vi "PTC-Create Queue Data.vi"(0 "state":T4, 5 "Params":T1, 9 "Acoustic System ID":string) -> (8 "data":T5, 15 "error out":errorcluster)   [LabVIEW 2020]
uses:
  Typedefs/PTC-Queue Data.ctl
  Common VIs/Typedefs/CAL-Stimulus.ctl
  Typedefs/PTC-Response.ctl
  Common VIs/Typedefs/CAL-Endpoint.ctl
  Typedefs/PTC-Parameters.ctl
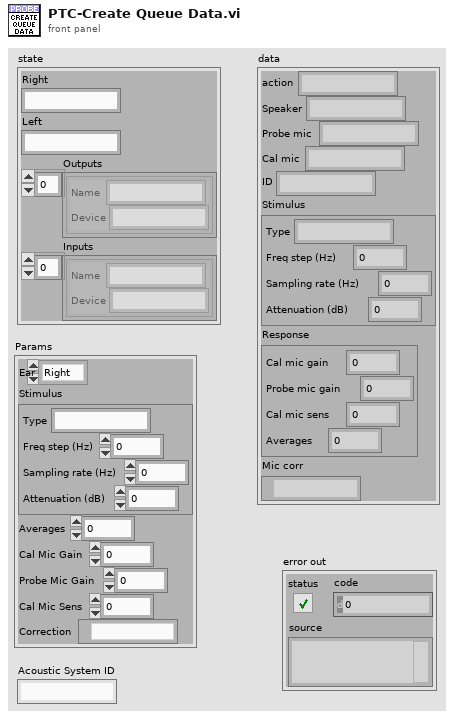
[diagram p1: front panel]
types:
  T1 = typedef "PTC-Parameters.ctl" = cluster{"Ear":enum16{"Right", "Left"}, "Stimulus":T2, "Averages":i32, "Cal Mic Gain":dbl, "Probe Mic Gain":dbl, "Cal Mic Sens":dbl, "Correction":path}
  T2 = typedef "CAL-Stimulus.ctl" = cluster{"Type":string, "Freq step (Hz)":dbl, "Sampling rate (Hz)":dbl, "Attenuation (dB)":dbl}
  T3 = typedef "CAL-Endpoint.ctl" = cluster{"Name":string, "Device":string}
  T4 = cluster{"Right":string, "Left":string, "Outputs":T3[], "Inputs":T3[]}
  T5 = typedef "PTC-Queue Data.ctl" = cluster{"action":string, "Speaker":string, "Probe mic":string, "Cal mic":string, "ID":string, "Stimulus":T2, "Response":T6, "Mic corr":path}
  T6 = typedef "PTC-Response.ctl" = cluster{"Cal mic gain":dbl, "Probe mic gain":dbl, "Cal mic sens":dbl, "Averages":i32}
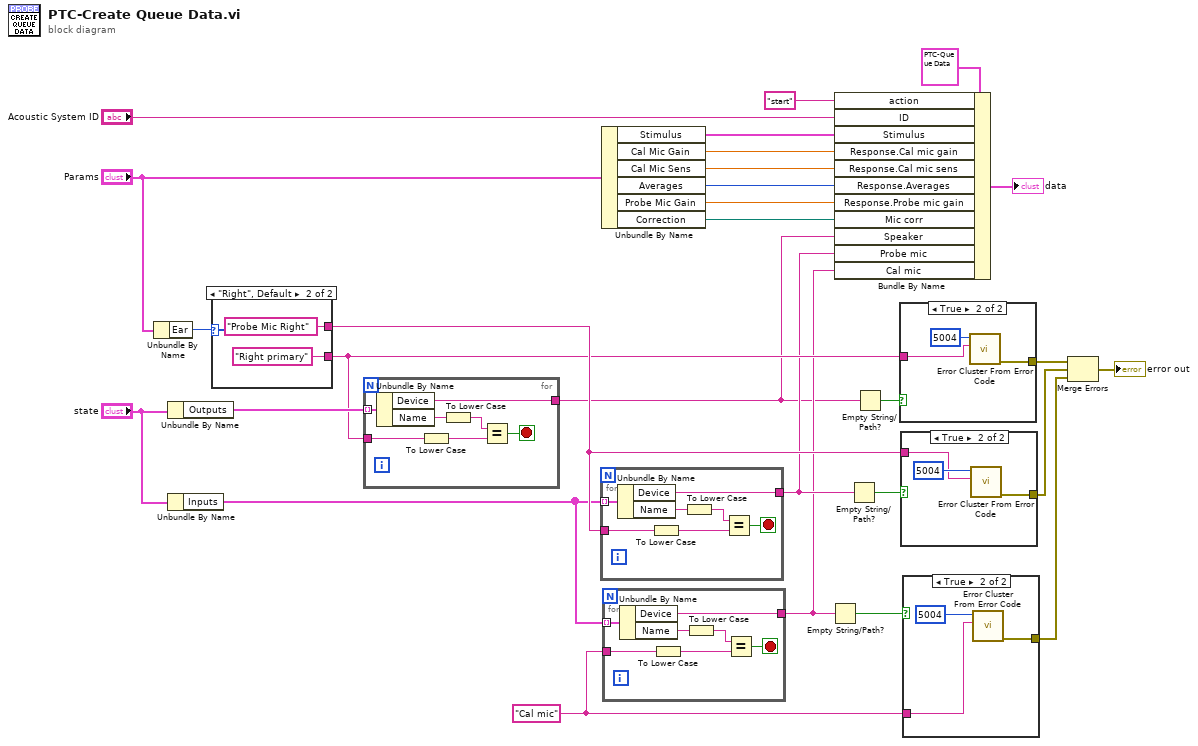
[diagram p0: block diagram]
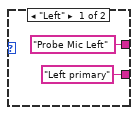
[diagram p3: hidden frame]
diagram:
  w4 = "Cal mic"
  n1 = Unbundle By Name("Params") -> ("Ear"=w24:enum16{"Right", "Left"})
  n2 = Unbundle By Name("state") -> ("Outputs"=w17:T3[])
  n3 = Unbundle By Name("state") -> ("Inputs"=w7:T3[])
  n4 = case shown="\"Right\", Default" w24 {
    tunnel: ["Left primary" "Right primary"] -> w9
    tunnel: ["Probe Mic Left" "Probe Mic Right"] -> w10
    frame "Left" {
    }
    frame "Right", Default {
    }
  }
  n5 = for {
    tunnel: w17 -> [w39] mode=indexing
    tunnel: [w36] -> w1
    tunnel: w9 -> [w35]
    stop <- w37 stop-if-true
    n6 = Unbundle By Name(w39) -> ("Device"=w36:string, "Name"=w38:string)
    n7 = To Lower Case(string=w35) -> (all lower case string=w33:string)
    n8 = To Lower Case(string=w38) -> (all lower case string=w34:string)
    n9 = Equal?(x=w34, y=w33) -> (x = y?=w37:bool)
  }
  n10 = for {
    tunnel: w7 -> [w46] mode=indexing
    tunnel: [w43] -> w8
    tunnel: w10 -> [w42]
    stop <- w44 stop-if-true
    n11 = Unbundle By Name(w46) -> ("Device"=w43:string, "Name"=w45:string)
    n12 = To Lower Case(string=w42) -> (all lower case string=w40:string)
    n13 = To Lower Case(string=w45) -> (all lower case string=w41:string)
    n14 = Equal?(x=w41, y=w40) -> (x = y?=w44:bool)
  }
  n15 = Unbundle By Name("Params") -> ("Stimulus"=w23:T2, "Cal Mic Gain"=w22:dbl, "Cal Mic Sens"=w21:dbl, "Averages"=w20:i32, "Probe Mic Gain"=w18:dbl, "Correction"=w2:path)
  n16 = for {
    tunnel: w7 -> [w53] mode=indexing
    tunnel: [w50] -> w5
    tunnel: w4 -> [w49]
    stop <- w51 stop-if-true
    n17 = Unbundle By Name(w53) -> ("Device"=w50:string, "Name"=w52:string)
    n18 = To Lower Case(string=w49) -> (all lower case string=w47:string)
    n19 = To Lower Case(string=w52) -> (all lower case string=w48:string)
    n20 = Equal?(x=w48, y=w47) -> (x = y?=w51:bool)
  }
  n21 = Empty String/Path?(string/path=w5) -> (empty?=w6:bool)
  n22 = Bundle By Name(cluster=T5 {"action"="", "Speaker"="", "Probe mic"="", "Cal mic"="", "ID"="", "Stimulus"={"Type"="", "Freq step (Hz)"=0.0, "Sampling rate (Hz)"=0.0, "Attenuation (dB)"=0.0}, "Response"={"Cal mic gain"=0.0, "Probe mic gain"=0.0, "Cal mic sens"=0.0, "Averages"=0}, "Mic corr"=path ""} ("data"), "action"="start", "ID"="Acoustic System ID", "Stimulus"=w23, "Response.Cal mic gain"=w22, "Response.Cal mic sens"=w21, "Response.Averages"=w20, "Response.Probe mic gain"=w18, "Mic corr"=w2, "Speaker"=w1, "Probe mic"=w8, "Cal mic"=w5) -> (→"data":T5)
  n23 = Empty String/Path?(string/path=w8) -> (empty?=w15:bool)
  n24 = Empty String/Path?(string/path=w1) -> (empty?=w16:bool)
  n25 = case shown="True" w16 {
    tunnel: w9 -> [_ w55]
    tunnel: [_ w54] -> w14
    frame False {
    }
    frame True {
      n26 = call <vilib>:"Error Cluster From Error Code.vi"("error message (\"\")"=w55, "error code (0)"=5004) -> ("error out"=w54:errorcluster)  [unwired: 7 in]
    }
  }
  n27 = case shown="True" w15 {
    tunnel: [_ w58] -> w13
    tunnel: w10 -> [_ w57]
    frame False {
    }
    frame True {
      n28 = call <vilib>:"Error Cluster From Error Code.vi"("error message (\"\")"=w57, "error code (0)"=5004) -> ("error out"=w58:errorcluster)  [unwired: 7 in]
    }
  }
  n29 = case shown="True" w6 {
    tunnel: [_ w61] -> w3
    tunnel: w4 -> [_ w60]
    frame False {
    }
    frame True {
      n30 = call <vilib>:"Error Cluster From Error Code.vi"("error message (\"\")"=w60, "error code (0)"=5004) -> ("error out"=w61:errorcluster)  [unwired: 7 in]
    }
  }
  n31 = Merge Errors(w14, w13, w3) -> (→"error out":errorcluster)
